vi "VLCPlayer.vi"(8 "stop ref in":refnum<vi>, 10 "movie folder":path, 11 "VLC Reference In":refnum<vi>) -> ()   [LabVIEW 2019]
panel:
  in  "VLCPlugin2":refnum<k7>(container)
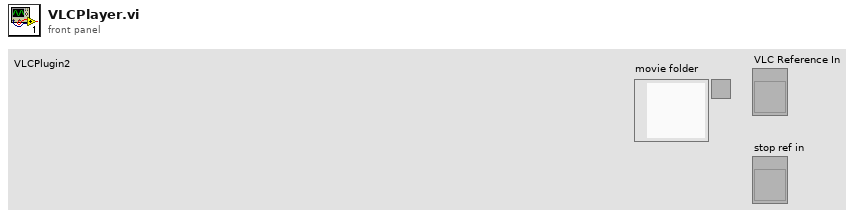
[diagram p1: front panel]
types:
  T1 = enum32{"Invalid", "Standard", "Closed", "Hidden", "Minimized", "Maximized"}
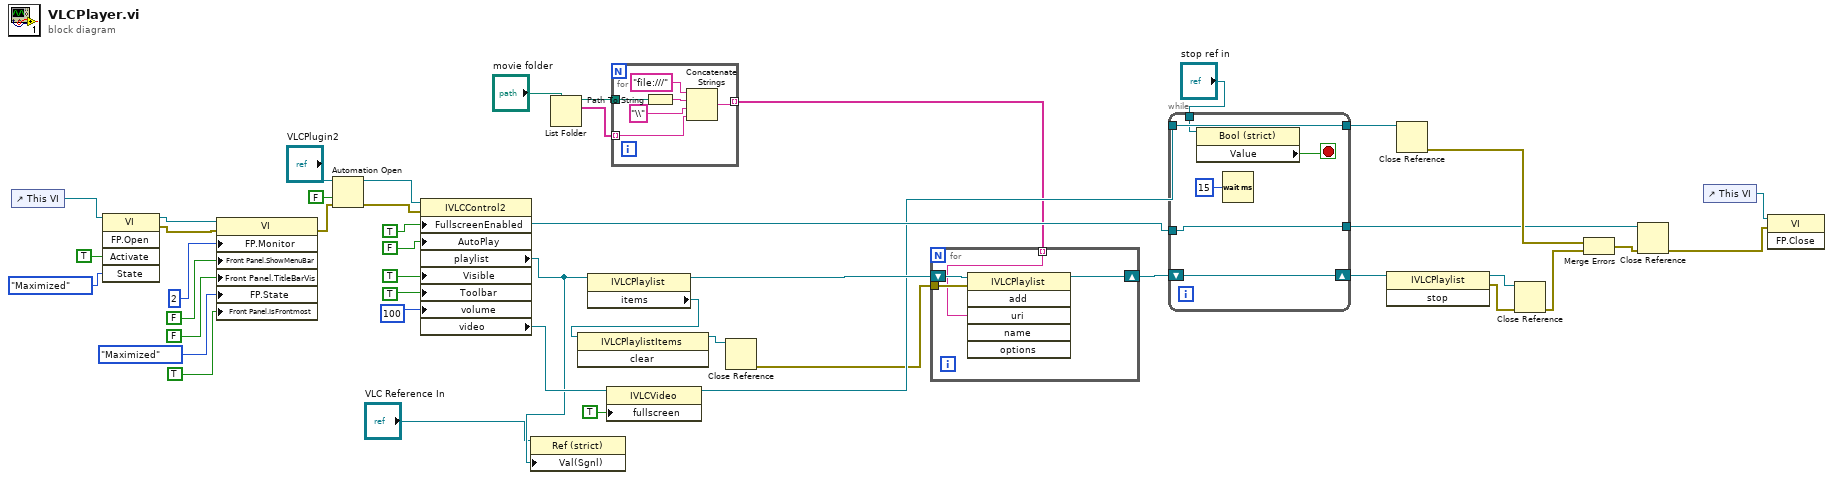
[diagram p0: block diagram]
diagram:
  n1 = control-ref of="This VI"() -> (w15:refnum<vi>)
  n2 = invoke class="VI" method="FP.Open"(reference=w15, "Activate"=TRUE ("Activate?"), "State"=T1."Maximized") -> (reference out=w17:refnum<vi>, error out=w16:errorcluster)  [unwired: 2 in, 3 out]
  n3 = property class="VI"(reference=w17, error in=w16, "FP.Monitor"=u16 2 ("Front Panel Window:Monitor"), "Front Panel.ShowMenuBar"=FALSE ("Front Panel Window:Show Menu Bar"), "Front Panel.TitleBarVis"=FALSE ("Front Panel Window:Title Bar Visible"), "FP.State"=T1."Maximized" ("Front Panel Window:State"), "Front Panel.IsFrontmost"=TRUE ("Front Panel Window:Is Frontmost")) -> (error out=w19:errorcluster)  [unwired: 1 out]
  n4 = Automation Open(error in (no error)=w19, Automation Refnum="VLCPlugin2", 9:FALSE ("open new instance (false)")) -> (Automation Refnum=w41:refnum<k7>, error out=w20:errorcluster)  [unwired: 1 in]
  n5 = property class="IVLCControl2"(reference=w41, error in=w20, "FullscreenEnabled"=TRUE, "AutoPlay"=FALSE, "Visible"=TRUE, "Toolbar"=TRUE ("Visible"), "volume"=100) -> (reference out=w44:refnum<k7>, "playlist"=w8:refnum<k7>, "video"=w33:refnum<k7>)  [unwired: 1 out]
  n6 = property class="Ref (strict)"(reference="VLC Reference In", "Val(Sgnl)"=w8) -> ()  [unwired: 1 in, 2 out]
  n7 = List Folder(path="movie folder") -> (path out=w4:path, filenames=w3:string[])  [unwired: 3 in, 2 out]
  n8 = property class="IVLCPlaylist"(reference=w8) -> (reference out=w37:refnum<k7>, "items"=w38:refnum<k7>)  [unwired: 1 in, 1 out]
  n9 = invoke class="IVLCPlaylistItems" method="clear"(reference=w38) -> (reference out=w40:refnum<k7>)  [unwired: 2 in, 2 out]
  n10 = property class="IVLCVideo"(reference=w33, "fullscreen"=TRUE) -> (reference out=w30:refnum<k7>)  [unwired: 1 in, 1 out]
  n11 = for {
    tunnel: w4 -> [w52]
    tunnel: w3 -> [w48] mode=indexing
    tunnel: [w49] -> w2 mode=indexing
    n12 = Path To String(path=w52) -> (string=w50:string)
    n13 = Concatenate Strings("file:///" ("string"), w50, "\\" ("string"), w48) -> (w49:string)
  }
  n14 = Close Reference(reference=w40) -> (error out=w1:errorcluster)  [unwired: 1 in]
  n15 = for {
    tunnel: w1 -> [w55]
    tunnel: w2 -> [w53] mode=indexing
    shift-right: [w54] -> w11
    shift-left: w37 -> [w56]
    n16 = invoke class="IVLCPlaylist" method="add"(reference=w56, error in=w55, "uri"=w53) -> (reference out=w54:refnum<k7>)  [unwired: 3 in, 5 out]
  }
  n17 = while {
    tunnel: w44 -> [w59]
    shift-right: [w61] -> w31
    shift-left: w11 -> [w61]
    tunnel: w30 -> [w60]
    tunnel: [w60] -> w29
    tunnel: [w59] -> w13
    tunnel: "stop ref in" -> [w57]
    stop <- w58 stop-if-true
    n18 = property class="Bool (strict)"(reference=w57) -> ("Value"=w58:bool)  [unwired: 1 in, 2 out]
    n19 = Wait (ms)(milliseconds to wait=u32 15) -> ()  [unwired: 1 out]
  }
  n20 = invoke class="IVLCPlaylist" method="stop"(reference=w31) -> (reference out=w39:refnum<k7>, error out=w28:errorcluster)  [unwired: 2 in, 1 out]
  n21 = Close Reference(reference=w29) -> (error out=w27:errorcluster)  [unwired: 1 in]
  n22 = Close Reference(reference=w39, error in (no error)=w28) -> (error out=w12:errorcluster)
  n23 = Merge Errors(w27, w12) -> (w26:errorcluster)
  n24 = Close Reference(reference=w13, error in (no error)=w26) -> (error out=w9:errorcluster)
  n25 = control-ref of="This VI"() -> (w10:refnum<vi>)
  n26 = invoke class="VI" method="FP.Close"(reference=w10, error in=w9) -> ()  [unwired: 1 in, 3 out]
